vi "H3C psw cable 10G QSFP+读写操作_old.vi"(6 "input_psw":u8[](array[numeric]) format="%.0x", 8 "input_data":u8[](array[numeric]) format="%.0x", 9 "input_mode":string(combo), 10 "Channel":u8 max=5 step=1, 11 "VISA":refnum<visa-resource-name>="COM6") -> (0 "123equal0?":bool, 1 "result":bool, 2 "message":string, 3 "data read":u8[](array[numeric]) format="%.0x")   [LabVIEW 2011]
panel:
  out "page3 128 Bytes":u8[](array[numeric]) format="%.0x"
  out "page2 128 Bytes":u8[](array[numeric]) format="%.0x"
  out "page1 128 Bytes":u8[](array[numeric]) format="%.0x"
  in  "address":u8
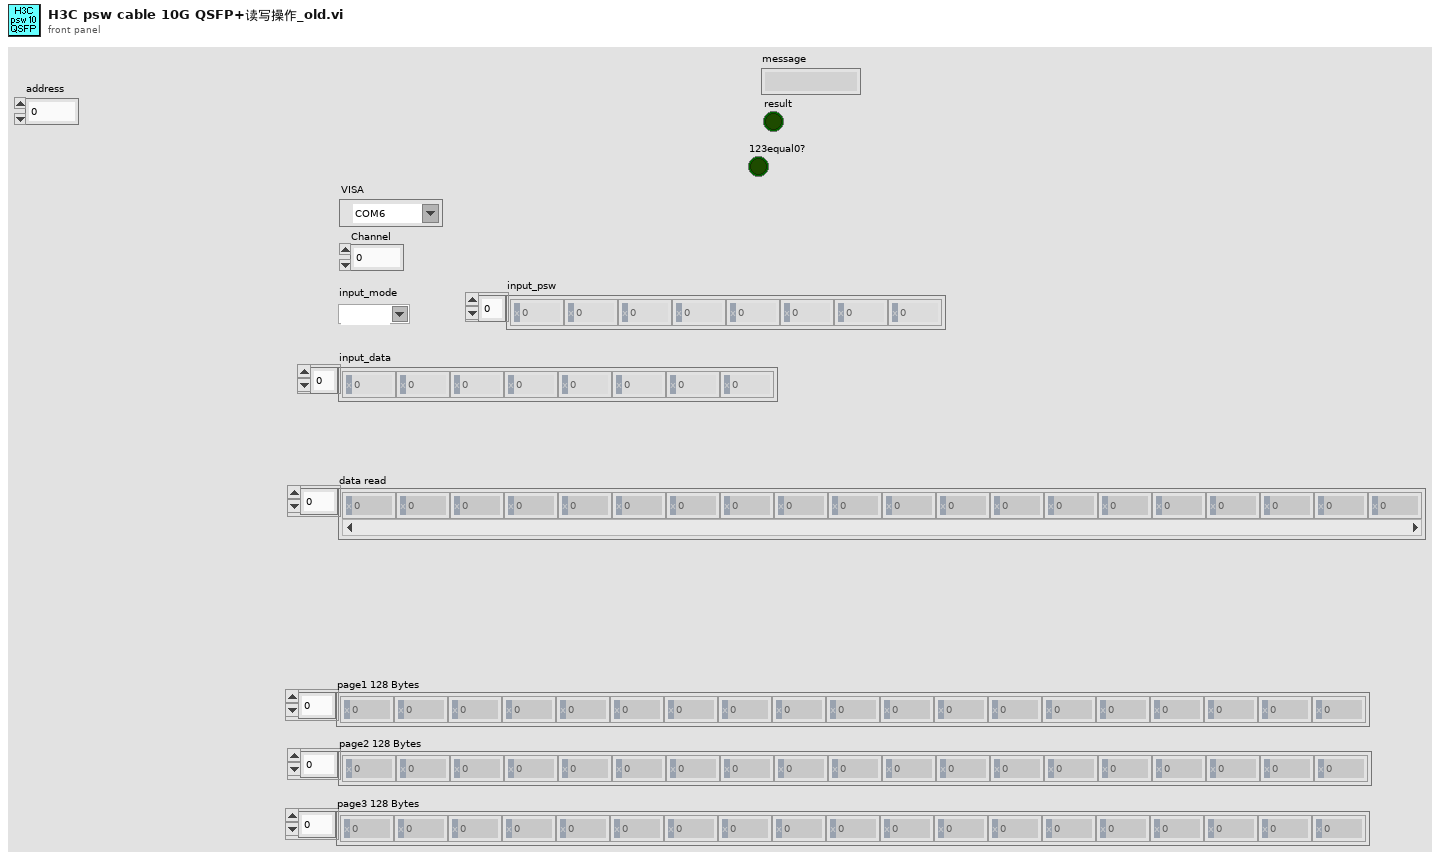
[diagram p1: front panel]
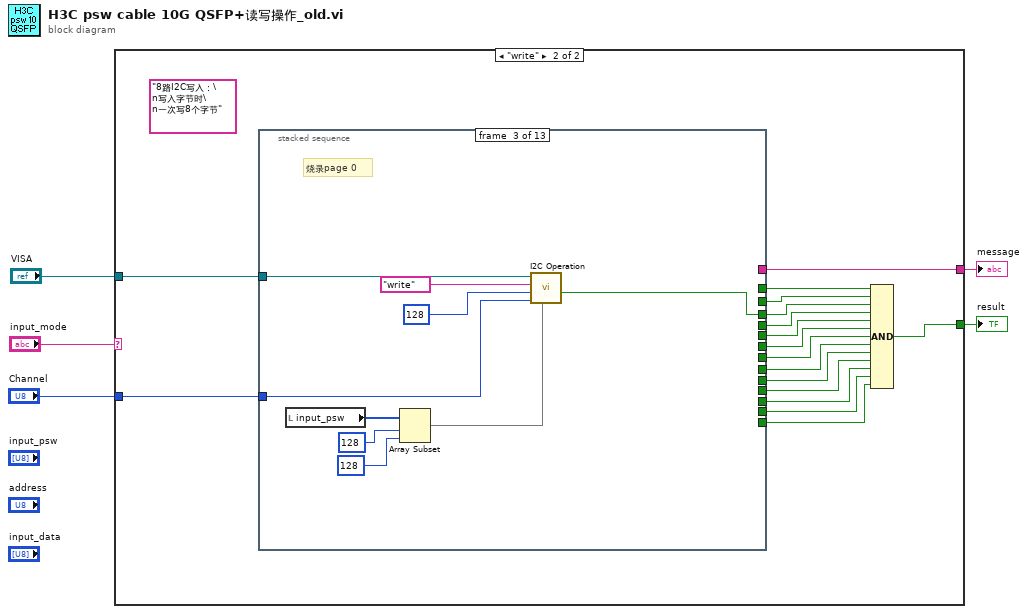
[diagram p0: block diagram]
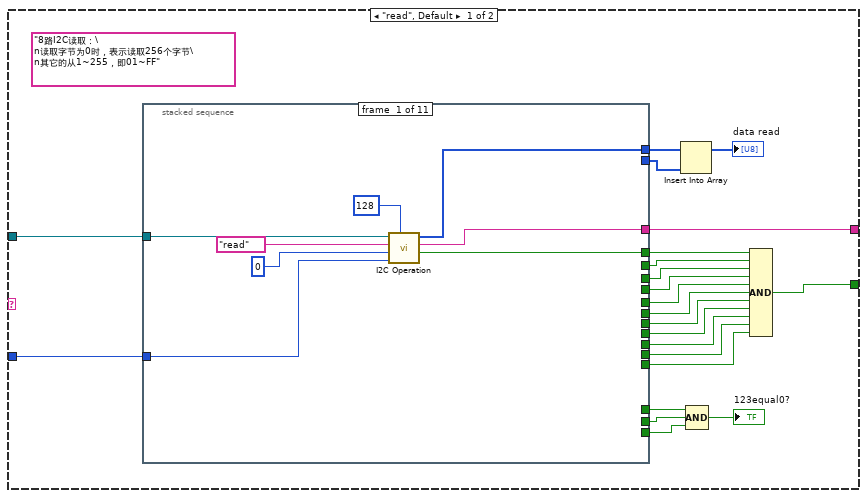
[diagram p2: hidden frame]
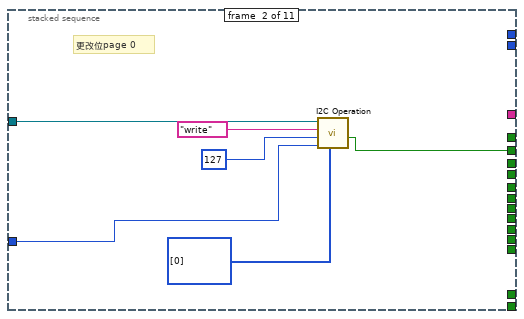
[diagram p3: hidden frame]
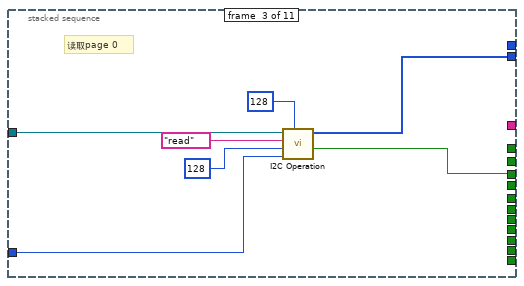
[diagram p4: hidden frame]
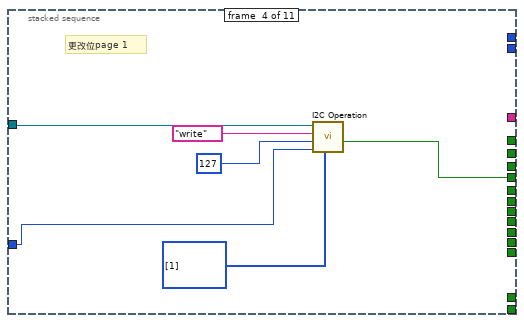
[diagram p5: hidden frame]
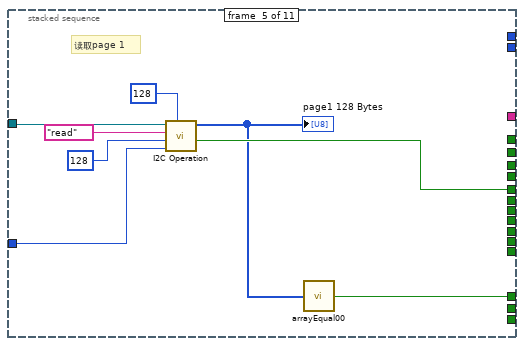
[diagram p6: hidden frame]
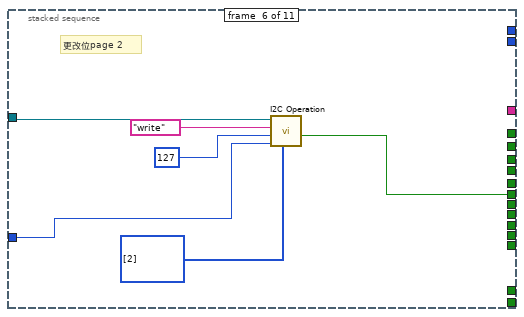
[diagram p7: hidden frame]
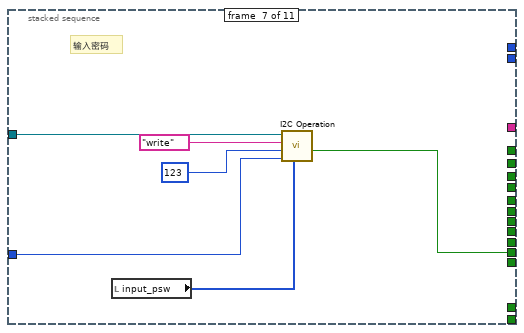
[diagram p8: hidden frame]
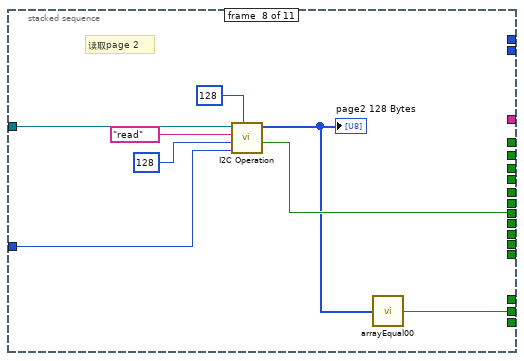
[diagram p9: hidden frame]
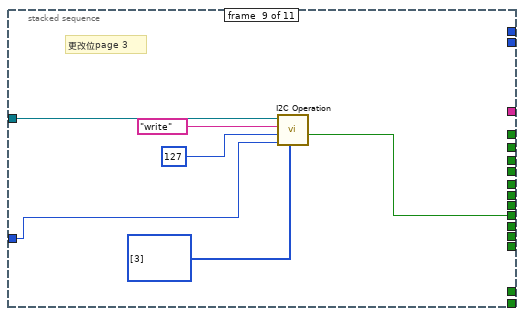
[diagram p10: hidden frame]
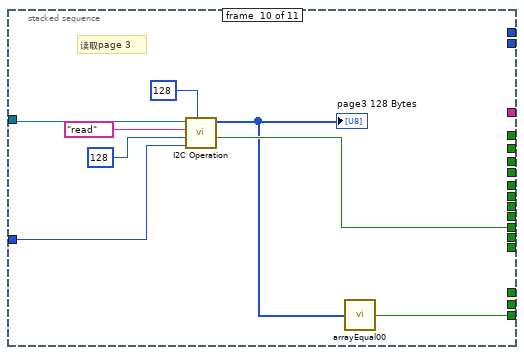
[diagram p11: hidden frame]
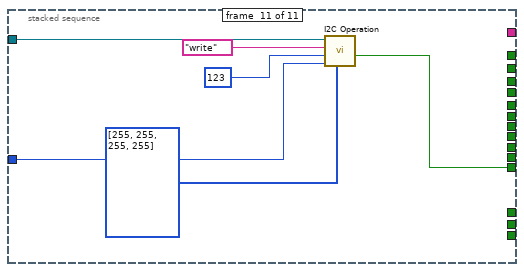
[diagram p12: hidden frame]
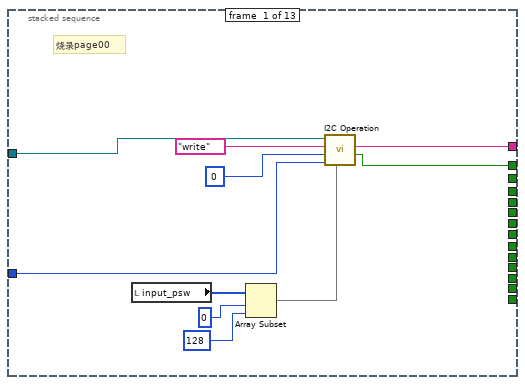
[diagram p13: hidden frame]
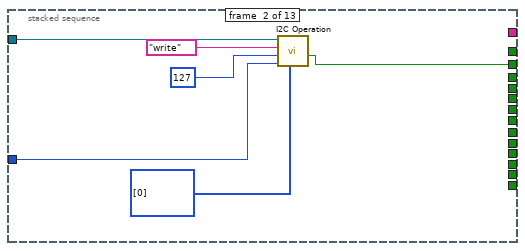
[diagram p14: hidden frame]
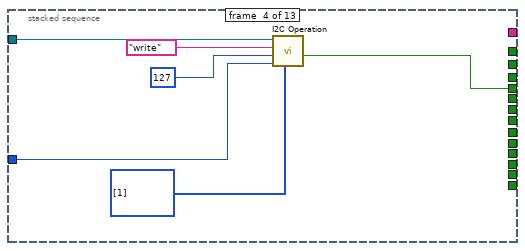
[diagram p15: hidden frame]
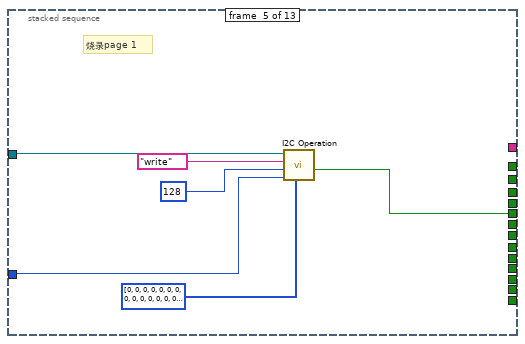
[diagram p16: hidden frame]
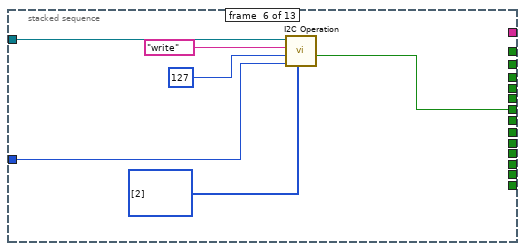
[diagram p17: hidden frame]
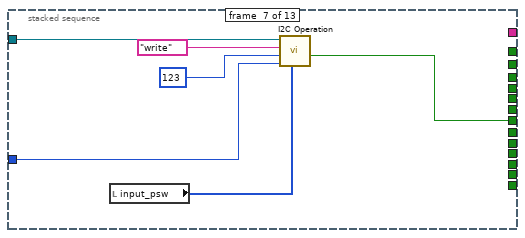
[diagram p18: hidden frame]
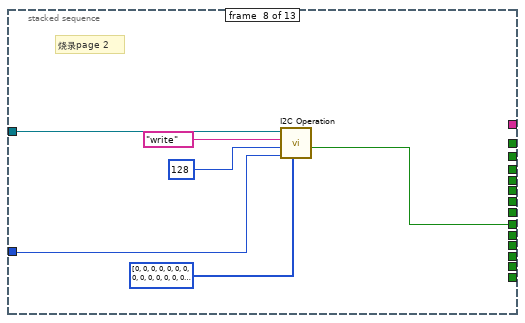
[diagram p19: hidden frame]
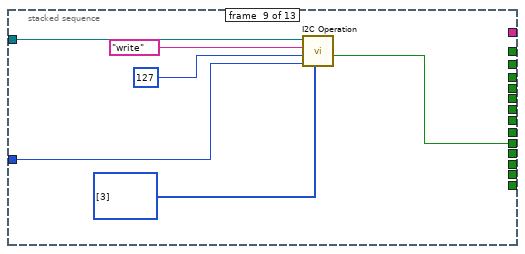
[diagram p20: hidden frame]
diagram:
  n1 = case shown="\"write\"" "input_mode" {
    tunnel: "VISA" -> [w27 w119]
    tunnel: "Channel" -> [w26 w118]
    tunnel: [w25 w117] -> w2
    tunnel: [w12 w103] -> w1
    frame "read", Default {
      (unwired) "8路I2C读取：\n读取字节为0时，表示读取256个字节\n其它的从1~255，即01~FF"
      n2 = stacked-sequence {
        tunnel: w27 -> [w35 w38 w48 w51 w59 w65 w71 w79 w85 w93 w100]
        tunnel: w26 -> [w31 w37 w44 w50 w58 w64 w70 w78 w84 w92 w99]
        tunnel: [w30 _ _ _ _ _ _ _ _ _ _] -> w25
        tunnel: [w29 _ _ _ _ _ _ _ _ _ _] -> w21
        tunnel: [w28 _ _ _ _ _ _ _ _ _ _] -> w24
        tunnel: [_ _ w43 _ _ _ _ _ _ _ _] -> w23
        tunnel: [_ w36 _ _ _ _ _ _ _ _ _] -> w20
        tunnel: [_ _ w42 _ _ _ _ _ _ _ _] -> w19
        tunnel: [_ _ _ w49 _ _ _ _ _ _ _] -> w18
        tunnel: [_ _ _ _ w57 _ _ _ _ _ _] -> w17
        tunnel: [_ _ _ _ _ w63 _ _ _ _ _] -> w16
        tunnel: [_ _ _ _ _ _ _ w77 _ _ _] -> w15
        tunnel: [_ _ _ _ _ _ _ _ w83 _ _] -> w14
        tunnel: [_ _ _ _ _ _ _ _ _ w91 _] -> w13
        tunnel: [_ _ _ _ _ _ w69 _ _ _ _] -> w11
        tunnel: [_ _ _ _ _ _ _ _ _ _ w97] -> w10
        tunnel: [_ _ _ _ w55 _ _ _ _ _ _] -> w9
        tunnel: [_ _ _ _ _ _ _ w76 _ _ _] -> w8
        tunnel: [_ _ _ _ _ _ _ _ _ w90 _] -> w7
        frame #0 {
          n3 = call "I2C Operation.vi"("size"=128, "Channel"=w31, "address"=u8 0, "mode"="read", "VISA"=w35) -> ("result"=w29:bool, "message"=w30:string, "Data Out"=w28:u8[])  [unwired: 4 in]
        }
        frame #1 {
          # "更改位page 0"
          n4 = call "I2C Operation.vi"("input_data"=u8[] [0], "Channel"=w37, "address"=u8 127, "mode"="write", "VISA"=w38) -> ("result"=w36:bool)  [unwired: 4 in, 2 out]
        }
        frame #2 {
          # "读取page 0"
          n5 = call "I2C Operation.vi"("size"=128, "Channel"=w44, "address"=u8 128, "mode"="read", "VISA"=w48) -> ("result"=w42:bool, "Data Out"=w43:u8[])  [unwired: 4 in, 1 out]
        }
        frame #3 {
          # "更改位page 1"
          n6 = call "I2C Operation.vi"("input_data"=u8[] [1], "Channel"=w50, "address"=u8 127, "mode"="write", "VISA"=w51) -> ("result"=w49:bool)  [unwired: 4 in, 2 out]
        }
        frame #4 {
          # "读取page 1"
          n7 = call "I2C Operation.vi"("size"=128, "Channel"=w58, "address"=u8 128, "mode"="read", "VISA"=w59) -> ("result"=w57:bool, "Data Out"=w56:u8[])  [unwired: 4 in, 1 out]
          "page1 128 Bytes" <- w56
          n8 = call "arrayEqual00.vi"("input"=w56) -> ("equal"=w55:bool)
        }
        frame #5 {
          # "更改位page 2"
          n9 = call "I2C Operation.vi"("input_data"=u8[] [2], "Channel"=w64, "address"=u8 127, "mode"="write", "VISA"=w65) -> ("result"=w63:bool)  [unwired: 4 in, 2 out]
        }
        frame #6 {
          # "输入密码"
          n10 = local read "input_psw"() -> (w72:u8[])
          n11 = call "I2C Operation.vi"("input_data"=w72, "Channel"=w70, "address"=u8 123, "mode"="write", "VISA"=w71) -> ("result"=w69:bool)  [unwired: 4 in, 2 out]
        }
        frame #7 {
          # "读取page 2"
          n12 = call "I2C Operation.vi"("size"=128, "Channel"=w78, "address"=u8 128, "mode"="read", "VISA"=w79) -> ("result"=w77:bool, "Data Out"=w75:u8[])  [unwired: 4 in, 1 out]
          "page2 128 Bytes" <- w75
          n13 = call "arrayEqual00.vi"("input"=w75) -> ("equal"=w76:bool)
        }
        frame #8 {
          # "更改位page 3"
          n14 = call "I2C Operation.vi"("input_data"=u8[] [3], "Channel"=w84, "address"=u8 127, "mode"="write", "VISA"=w85) -> ("result"=w83:bool)  [unwired: 4 in, 2 out]
        }
        frame #9 {
          # "读取page 3"
          n15 = call "I2C Operation.vi"("size"=128, "Channel"=w92, "address"=u8 128, "mode"="read", "VISA"=w93) -> ("result"=w91:bool, "Data Out"=w89:u8[])  [unwired: 4 in, 1 out]
          "page3 128 Bytes" <- w89
          n16 = call "arrayEqual00.vi"("input"=w89) -> ("equal"=w90:bool)
        }
        frame #10 {
          n17 = call "I2C Operation.vi"("input_data"=u8[] [255, 255, 255, 255], "Channel"=w99, "address"=u8 123, "mode"="write", "VISA"=w100) -> ("result"=w97:bool)  [unwired: 4 in, 2 out]
        }
      }
      n18 = Insert Into Array(array=w24, new element=w23) -> (→"data read":u8[])  [unwired: 1 in]
      n19 = Compound Arithmetic op=AND(w9, w8, w7) -> (→"123equal0?":bool)
      n20 = Compound Arithmetic op=AND(w21, w20, w19, w18, w17, w16, w15, w14, w13, w11, w10) -> (w12:bool)
    }
    frame "write" {
      (unwired) "8路I2C写入：\n写入字节时\n一次写8个字节"
      n21 = stacked-sequence {
        tunnel: w119 -> [w129 w135 w144 w146 w153 w159 w165 w171 w176 w183 w190 w196 w202]
        tunnel: w118 -> [w127 w133 w142 w147 w152 w160 w166 w170 w177 w182 w189 w195 w201]
        tunnel: [w126 _ _ _ _ _ _ _ _ _ _ _ _] -> w117
        tunnel: [w125 _ _ _ _ _ _ _ _ _ _ _ _] -> w116
        tunnel: [_ w130 _ _ _ _ _ _ _ _ _ _ _] -> w115
        tunnel: [_ _ w140 _ _ _ _ _ _ _ _ _ _] -> w114
        tunnel: [_ _ _ w145 _ _ _ _ _ _ _ _ _] -> w113
        tunnel: [_ _ _ _ w151 _ _ _ _ _ _ _ _] -> w112
        tunnel: [_ _ _ _ _ w157 _ _ _ _ _ _ _] -> w111
        tunnel: [_ _ _ _ _ _ w163 _ _ _ _ _ _] -> w110
        tunnel: [_ _ _ _ _ _ _ w169 _ _ _ _ _] -> w109
        tunnel: [_ _ _ _ _ _ _ _ w175 _ _ _ _] -> w108
        tunnel: [_ _ _ _ _ _ _ _ _ w181 _ _ _] -> w107
        tunnel: [_ _ _ _ _ _ _ _ _ _ w187 _ _] -> w106
        tunnel: [_ _ _ _ _ _ _ _ _ _ _ w193 _] -> w105
        tunnel: [_ _ _ _ _ _ _ _ _ _ _ _ w199] -> w104
        frame #0 {
          # "烧录page00"
          n22 = local read "input_psw"() -> (w123:u8[])
          n23 = Array Subset(array=w123, index=0 ("索引"), length=128 ("长度")) -> (w121:u8[])
          n24 = call "I2C Operation.vi"("input_data"=w121, "Channel"=w127, "address"=u8 0, "mode"="write", "VISA"=w129) -> ("result"=w125:bool, "message"=w126:string)  [unwired: 4 in, 1 out]
        }
        frame #1 {
          n25 = call "I2C Operation.vi"("input_data"=u8[] [0], "Channel"=w133, "address"=u8 127, "mode"="write", "VISA"=w135) -> ("result"=w130:bool)  [unwired: 4 in, 2 out]
        }
        frame #2 {
          # "烧录page 0"
          n26 = local read "input_psw"() -> (w139:u8[])
          n27 = Array Subset(array=w139, index=128 ("索引"), length=128 ("长度")) -> (w136:u8[])
          n28 = call "I2C Operation.vi"("input_data"=w136, "Channel"=w142, "address"=u8 128, "mode"="write", "VISA"=w144) -> ("result"=w140:bool)  [unwired: 4 in, 2 out]
        }
        frame #3 {
          n29 = call "I2C Operation.vi"("input_data"=u8[] [1], "Channel"=w147, "address"=u8 127, "mode"="write", "VISA"=w146) -> ("result"=w145:bool)  [unwired: 4 in, 2 out]
        }
        frame #4 {
          # "烧录page 1"
          n30 = call "I2C Operation.vi"("input_data"=u8[] [0, 0, 0, 0, 0, 0, 0, 0, 0, 0, 0, 0, 0, 0, 0, 0, 0, 0, 0, 0, 0, 0, 0, 0, 0, 0, 0, 0, 0, 0, 0, 0, 0, 0, 0, 0, 0, 0, 0, 0, 0, 0, 0, 0, 0, 0, 0, 0, 0, 0, 0, 0, 0, 0, 0, 0, 0, 0, 0, 0, 0, 0, 0, 0, 0, 0, 0, 0, 0, 0, 0, 0, 0, 0, 0, 0, 0, 0, 0, 0, 0, 0, 0, 0, 0, 0, 0, 0, 0, 0, 0, 0, 0, 0, 0, 0, 0, 0, 0, 0, 0, 0, 0, 0, 0, 0, 0, 0, 0, 0, 0, 0, 0, 0, 0, 0, 0, 0, 0, 0, 0, 0, 0, 0, 0, 0, 0, 0], "Channel"=w152, "address"=u8 128, "mode"="write", "VISA"=w153) -> ("result"=w151:bool)  [unwired: 4 in, 2 out]
        }
        frame #5 {
          n31 = call "I2C Operation.vi"("input_data"=u8[] [2], "Channel"=w160, "address"=u8 127, "mode"="write", "VISA"=w159) -> ("result"=w157:bool)  [unwired: 4 in, 2 out]
        }
        frame #6 {
          n32 = local read "input_psw"() -> (w164:u8[])
          n33 = call "I2C Operation.vi"("input_data"=w164, "Channel"=w166, "address"=u8 123, "mode"="write", "VISA"=w165) -> ("result"=w163:bool)  [unwired: 4 in, 2 out]
        }
        frame #7 {
          # "烧录page 2"
          n34 = call "I2C Operation.vi"("input_data"=u8[] [0, 0, 0, 0, 0, 0, 0, 0, 0, 0, 0, 0, 0, 0, 0, 0, 0, 0, 0, 0, 0, 0, 0, 0, 0, 0, 0, 0, 0, 0, 0, 0, 0, 0, 0, 0, 0, 0, 0, 0, 0, 0, 0, 0, 0, 0, 0, 0, 0, 0, 0, 0, 0, 0, 0, 0, 0, 0, 0, 0, 0, 0, 0, 0, 0, 0, 0, 0, 0, 0, 0, 0, 0, 0, 0, 0, 0, 0, 0, 0, 0, 0, 0, 0, 0, 0, 0, 0, 0, 0, 0, 0, 0, 0, 0, 0, 0, 0, 0, 0, 0, 0, 0, 0, 0, 0, 0, 0, 0, 0, 0, 0, 0, 0, 0, 0, 0, 0, 0, 0, 0, 0, 0, 0, 0, 0, 0, 0], "Channel"=w170, "address"=u8 128, "mode"="write", "VISA"=w171) -> ("result"=w169:bool)  [unwired: 4 in, 2 out]
        }
        frame #8 {
          n35 = call "I2C Operation.vi"("input_data"=u8[] [3], "Channel"=w177, "address"=u8 127, "mode"="write", "VISA"=w176) -> ("result"=w175:bool)  [unwired: 4 in, 2 out]
        }
        frame #9 {
          # "烧录page 3"
          n36 = call "I2C Operation.vi"("input_data"=u8[] [0, 0, 0, 0, 0, 0, 0, 0, 0, 0, 0, 0, 0, 0, 0, 0, 0, 0, 0, 0, 0, 0, 0, 0, 0, 0, 0, 0, 0, 0, 0, 0, 0, 0, 0, 0, 0, 0, 0, 0, 0, 0, 0, 0, 0, 0, 0, 0, 0, 0, 0, 0, 0, 0, 0, 0, 0, 0, 0, 0, 0, 0, 0, 0, 0, 0, 0, 0, 0, 0, 0, 0, 0, 0, 0, 0, 0, 0, 0, 0, 0, 0, 0, 0, 0, 0, 0, 0, 0, 0, 0, 0, 0, 0, 0, 0, 0, 0, 0, 0, 0, 0, 0, 0, 0, 0, 0, 0, 0, 0, 0, 0, 0, 0, 0, 0, 0, 0, 0, 0, 0, 0, 0, 0, 0, 0, 0, 0], "Channel"=w182, "address"=u8 128, "mode"="write", "VISA"=w183) -> ("result"=w181:bool)  [unwired: 4 in, 2 out]
        }
        frame #10 {
          n37 = call "I2C Operation.vi"("input_data"=u8[] [0], "Channel"=w189, "address"=u8 127, "mode"="write", "VISA"=w190) -> ("result"=w187:bool)  [unwired: 4 in, 2 out]
        }
        frame #11 {
          n38 = call "I2C Operation.vi"("input_data"=u8[] [226, 23, 130, 37], "Channel"=w195, "address"=u8 123, "mode"="write", "VISA"=w196) -> ("result"=w193:bool)  [unwired: 4 in, 2 out]
        }
        frame #12 {
          n39 = call "I2C Operation.vi"("input_data"=u8[] [255, 255, 255, 255], "Channel"=w201, "address"=u8 123, "mode"="write", "VISA"=w202) -> ("result"=w199:bool)  [unwired: 4 in, 2 out]
        }
      }
      n40 = Compound Arithmetic op=AND(w116, w115, w114, w113, w112, w111, w110, w109, w108, w107, w106, w105, w104) -> (w103:bool)
    }
  }
  "message" <- w2
  "result" <- w1
